vi "例4-3.vi"() -> ()   [LabVIEW 2019]
panel:
  out "N!":dbl
  in  "N":dbl=5.0
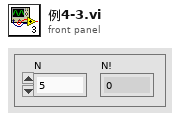
[diagram p1: front panel]
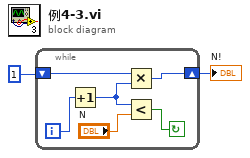
[diagram p0: block diagram]
diagram:
  n1 = while {
    shift-right: [w7] -> w1
    shift-left: 1 -> [w6]
    i -> [w8]
    stop <- w4 continue-if-true
    n2 = Increment(x=w8) -> (x+1=w5:i32)
    n3 = Multiply(x=w6, y=w5) -> (x*y=w7:i32)
    n4 = Less?(x=w5, y="N") -> (x < y?=w4:bool)
  }
  "N!" <- w1
